vi "Read Config.vi"(8 "error in (no error)":errorcluster, 11 "JsonReportPlugin in":refnum<class "JsonReportPlugin.lvclass">) -> (0 "error out":errorcluster, 2 "Config":variant, 3 "JsonReportPlugin out":refnum<class "JsonReportPlugin.lvclass">)   [LabVIEW 2015, in "JsonReportPlugin.lvclass"]
uses:
  JsonReportPlugin.lvclass
  JsonReportPlugin.lvclass/JsonReportPlugin.ctl
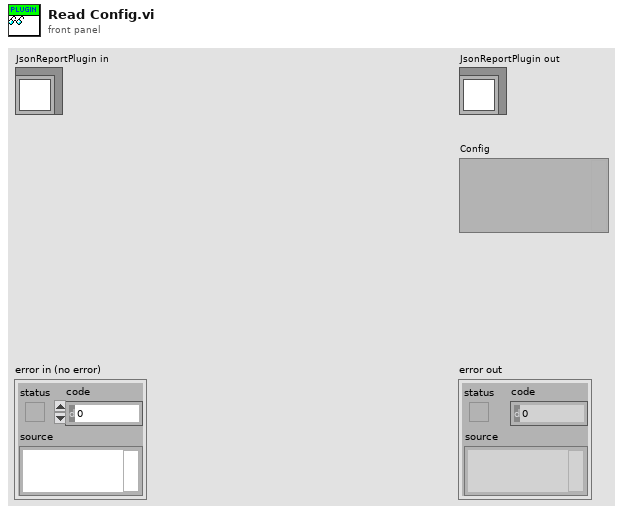
[diagram p1: front panel]
types:
  T1 = cluster{"Enable":bool, "Report Folder":string, "Include SN":bool, "Include Timestamp":bool, "Include Result":bool}
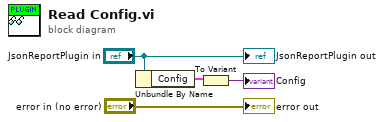
[diagram p0: block diagram]
diagram:
  n1 = Unbundle By Name("JsonReportPlugin in") -> ("Config"=w2:T1)
  n2 = To Variant(anything=w2) -> (Variant=→"Config":variant)
  "error out" <- "error in (no error)"
  "JsonReportPlugin out" <- "JsonReportPlugin in"
